vi "CRYSave Wave File.vi"(6 "Channel":u32=1, 8 "Wave Data In":sgl[](array[numeric]), 9 "Sampling Bit":u32=16, 10 "Sampling Freq":u32=44100, 11 "Wave File Path In":path) -> (0 "Error Out(0-OK)":u32)   [LabVIEW 2013]
uses:
  CRYSound.dll
panel:
  out "Waveform Graph":sgl[](graph)
  # "Save Wave File."
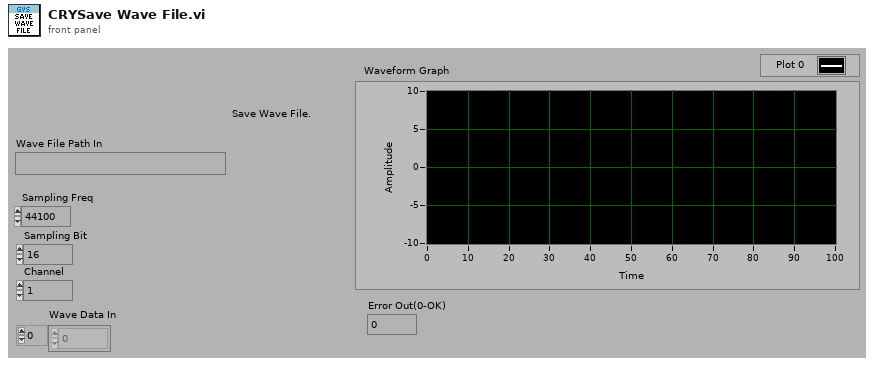
[diagram p1: front panel]
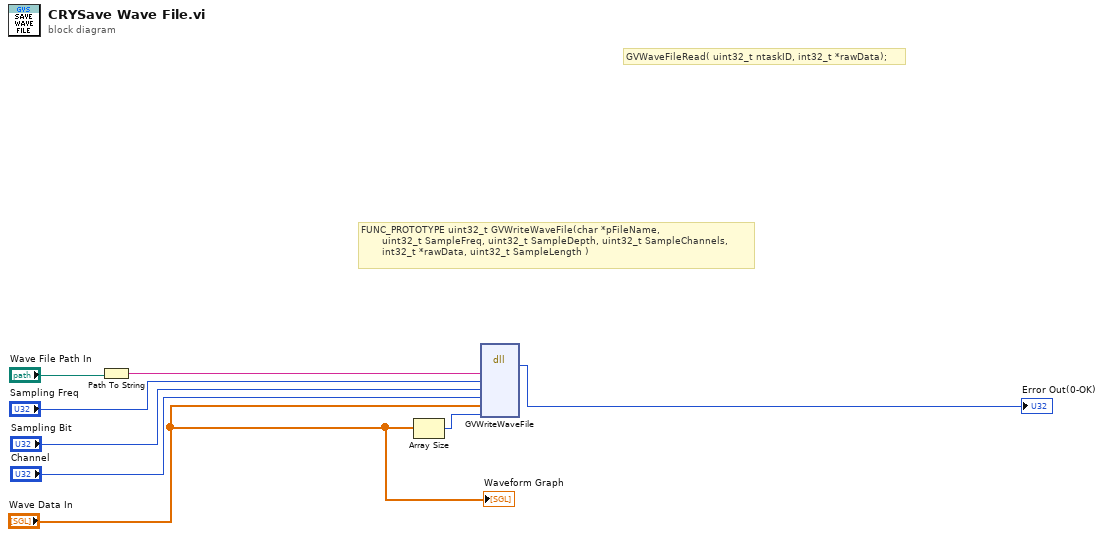
[diagram p0: block diagram]
diagram:
  # "FUNC_PROTOTYPE uint32_t GVWriteWaveFile(char *pFileName,\n\t\t\t\t\t\t uint32_t SampleFreq, uint32_t SampleDepth, uint32_t SampleChannels,\n\t\t\t\t\t\t int32_t *rawData, uint32_t SampleLength )"
  # "GVWaveFileRead( uint32_t ntaskID, int32_t *rawData);"
  n1 = Path To String(path="Wave File Path In") -> (string=w8:string)
  n2 = Array Size(array="Wave Data In") -> (size(s)=w2:i32)
  n3 = dll-call lib="D:/LabView_Project/CRY6181/CRYSound.dll" fn="GVWriteWaveFile"("WaveFileName"=w8, "SampleFreq"="Sampling Freq", "BitDepth"="Sampling Bit", "nChannels"="Channel", "Data"="Wave Data In", "SampleLength"=w2) -> ("return type"=→"Error Out(0-OK)":u32)  [unwired: 9 in, 2 out]
  "Waveform Graph" <- "Wave Data In"
